vi "Read Allow Saccades.vi"(8 "error in (no error)":errorcluster, 11 "TrialBasedExperiment in":refnum<class "TrialBasedExperiment.lvclass">) -> (0 "error out":errorcluster, 2 "Allow Saccades":bool, 3 "TrialBasedExperiment out":refnum<class "TrialBasedExperiment.lvclass">)   [LabVIEW 2014, in "AcquisitionCoreObjects.lvlib" / "TrialBasedExperiment.lvclass"]
uses:
  TrialBasedExperiment.lvclass
  TrialBasedExperiment.lvclass/TrialBasedExperiment.ctl
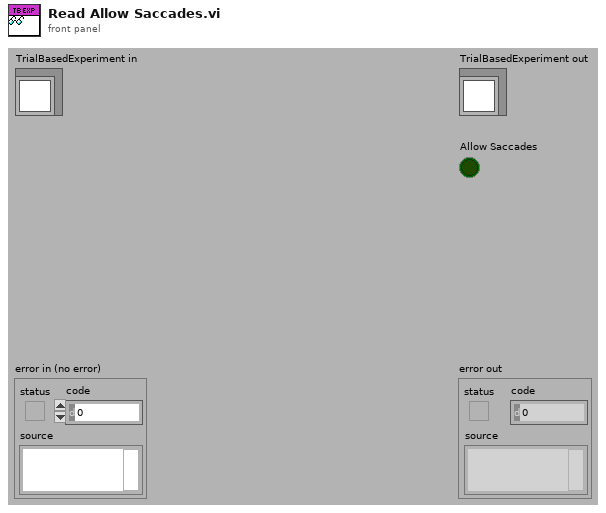
[diagram p1: front panel]
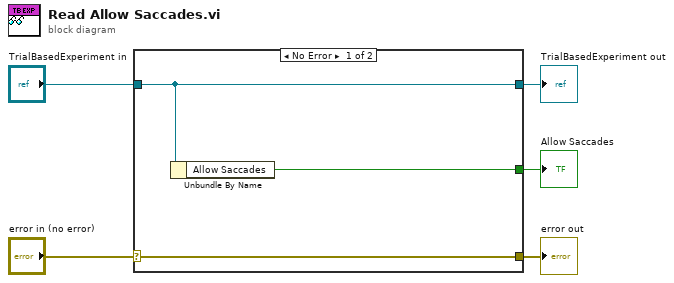
[diagram p0: block diagram]
diagram:
  n1 = case shown="No Error" "error in (no error)" {
    selector: "error in (no error)" -> [w8 w9]
    tunnel: [w8 w9] -> w4
    tunnel: [w7 w10] -> w2
    tunnel: "TrialBasedExperiment in" -> [w7 w10]
    tunnel: [w6 _] -> w1
    frame No Error {
      n2 = Unbundle By Name(w7) -> ("Allow Saccades"=w6:bool)
    }
    frame Error {
    }
  }
  "error out" <- w4
  "TrialBasedExperiment out" <- w2
  "Allow Saccades" <- w1
